vi "Licznik Symetralnej.vi"(2 "error in":errorcluster, 3 "Punkt 2":dbl[](array[numeric]), 4 "Punkt 1":dbl[](array[numeric])) -> (0 "error out":errorcluster, 1 "równanie prostej":dbl[](array[numeric]))   [LabVIEW 2016]
doc: "To vi przyjumje dwa punkty w przetrzeni 2D w układzie kartezjańskim i zwraca wartości A, B , C równania prostej Ax+By+C=0"
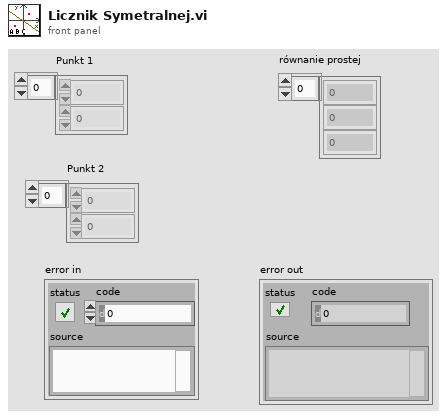
[diagram p1: front panel]
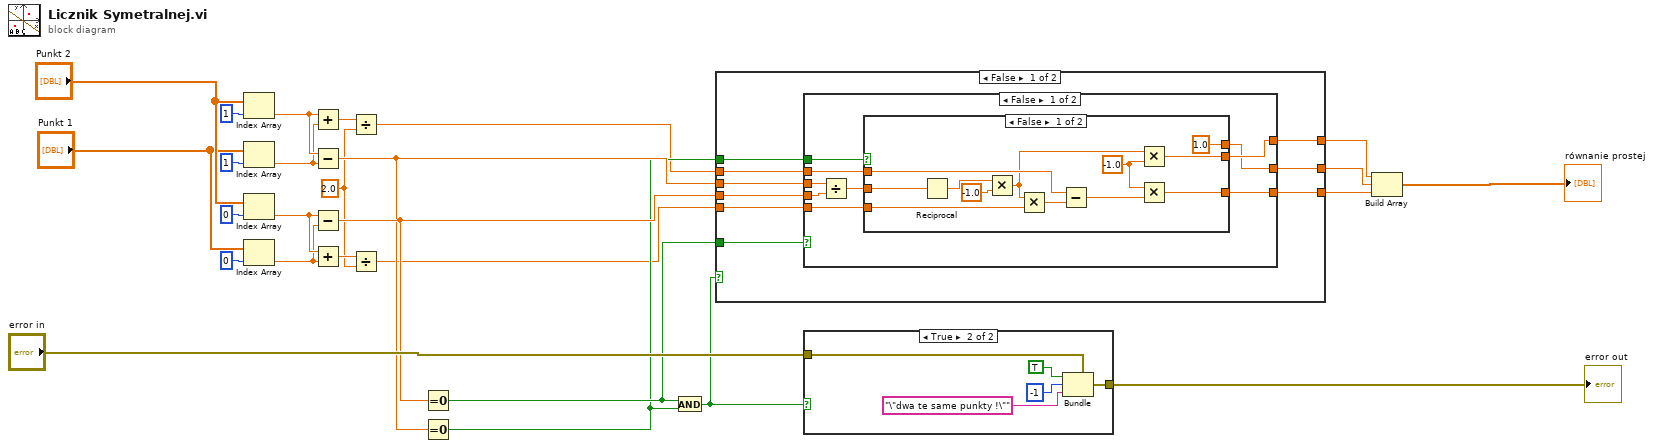
[diagram p0: block diagram]
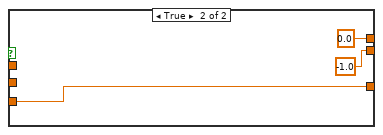
[diagram p2: hidden frame]
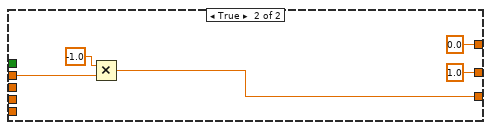
[diagram p3: hidden frame]
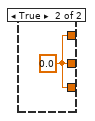
[diagram p4: hidden frame]
diagram:
  w6 = 2.0 ("y")
  n1 = Index Array(array="Punkt 2", index=1) -> (element=w12:dbl)
  n2 = Index Array(array="Punkt 1", index=1) -> (element=w11:dbl)
  n3 = Index Array(array="Punkt 2", index=0) -> (element=w10:dbl)
  n4 = Index Array(array="Punkt 1", index=0) -> (element=w9:dbl)
  n5 = Add(x=w12, y=w11) -> (x+y=w7:dbl)
  n6 = Subtract(x=w12, y=w11) -> (x-y=w16:dbl)
  n7 = Subtract(x=w10, y=w9) -> (x-y=w17:dbl)
  n8 = Add(x=w10, y=w9) -> (x+y=w8:dbl)
  n9 = Divide(x=w7, y=w6) -> (x/y=w5:dbl)
  n10 = Divide(x=w8, y=w6) -> (x/y=w4:dbl)
  n11 = Equal To 0?(x=w17) -> (x = 0?=w15:bool)
  n12 = Equal To 0?(x=w16) -> (x = 0?=w14:bool)
  n13 = And(x=w15, y=w14) -> (x .and. y?=w19:bool)
  n14 = case shown="False" w19 {
    tunnel: [w27 w65] -> w18
    tunnel: [w29 w65] -> w3
    tunnel: w17 -> [w32 _]
    tunnel: w16 -> [w33 _]
    tunnel: w15 -> [w35 _]
    tunnel: w14 -> [w34 _]
    tunnel: w5 -> [w31 _]
    tunnel: w4 -> [w30 _]
    tunnel: [w28 w65] -> w2
    frame False {
      n15 = case shown="False" w35 {
        tunnel: w32 -> [w43 _]
        tunnel: w33 -> [w44 _]
        tunnel: w34 -> [w42 _]
        tunnel: [w40 0.0] -> w27
        tunnel: [w39 w60] -> w29
        tunnel: w31 -> [w38 w61]
        tunnel: w30 -> [w37 _]
        tunnel: [w36 1.0] -> w28
        frame False {
          n16 = Divide(x=w44, y=w43) -> (x/y=w41:dbl)
          n17 = case shown="False" w42 {
            tunnel: w41 -> [w56 _]
            tunnel: [w45 -1.0] -> w40
            tunnel: [w48 w59] -> w39
            tunnel: w38 -> [w55 _]
            tunnel: w37 -> [w54 w59]
            tunnel: [1.0 0.0] -> w36
            frame False {
              w47 = -1.0
              n18 = Reciprocal(x=w56) -> (1/x=w50:dbl)
              n19 = Multiply(x=w50, y=-1.0) -> (x*y=w46:dbl)
              n20 = Multiply(x=w46, y=w54) -> (x*y=w53:dbl)
              n21 = Subtract(x=w55, y=w53) -> (x-y=w49:dbl)
              n22 = Multiply(x=w46, y=w47) -> (x*y=w45:dbl)
              n23 = Multiply(x=w47, y=w49) -> (x*y=w48:dbl)
            }
            frame True {
            }
          }
        }
        frame True {
          n24 = Multiply(x=-1.0, y=w61) -> (x*y=w60:dbl)
        }
      }
    }
    frame True {
      w65 = 0.0
    }
  }
  n25 = case shown="True" w19 {
    tunnel: [w66 w68] -> w21
    tunnel: "error in" -> [w66 w71]
    frame False {
    }
    frame True {
      n26 = Bundle(cluster=w71, "status"=TRUE, "code"=-1, "source"="\"dwa te same punkty !\"") -> (w68:errorcluster)
    }
  }
  "error out" <- w21
  n27 = Build Array(w18, w2, w3) -> (→"równanie prostej":dbl[])
